vi "test Deploy with Module Already Reserved.vi"(8 "error in (no error)":errorcluster, 11 "TestCase in":refnum<class "SLSC Switch System Tests.lvclass">) -> (0 "error out":errorcluster, 3 "TestCase out":refnum<class "SLSC Switch System Tests.lvclass">)   [LabVIEW 2019, in "SLSC Switch System Tests.lvclass"]
uses:
  SLSC Switch System Tests.lvclass
  <vilib>/addons/_JKI Toolkits/VI Tester/TestCase.llb/TestCase.lvclass
  <vilib>/NI/VeriStand Custom Device Testing Tools/VeriStandTestCase/VeriStandTestCase.lvclass
  <vilib>/SLSC/SLSC.lvlib
  <vilib>/SLSC/Initialize Session with Devices.vi
  <vilib>/SLSC/Close Session.vi
  C:/Dev/GitHub/niveristand-custom-device-testing-tools/VeriStandTestCase/VeriStandTestCase.lvclass
  C:/Program Files (x86)/National Instruments/LabVIEW 2019/vi.lib/addons/_JKI Toolkits/VI Tester/TestCase.llb/TestCase.lvclass
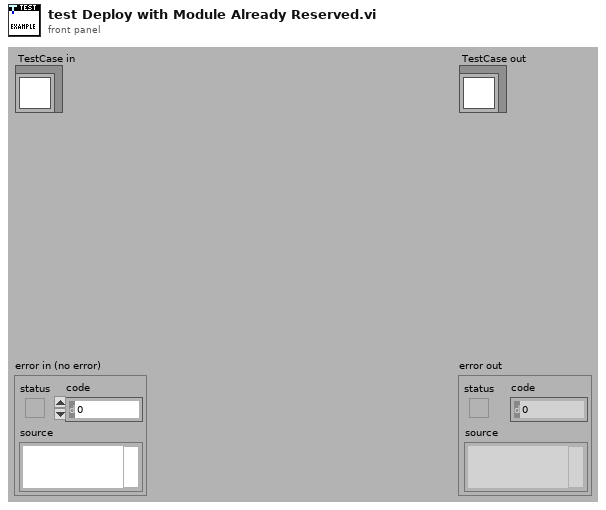
[diagram p1: front panel]
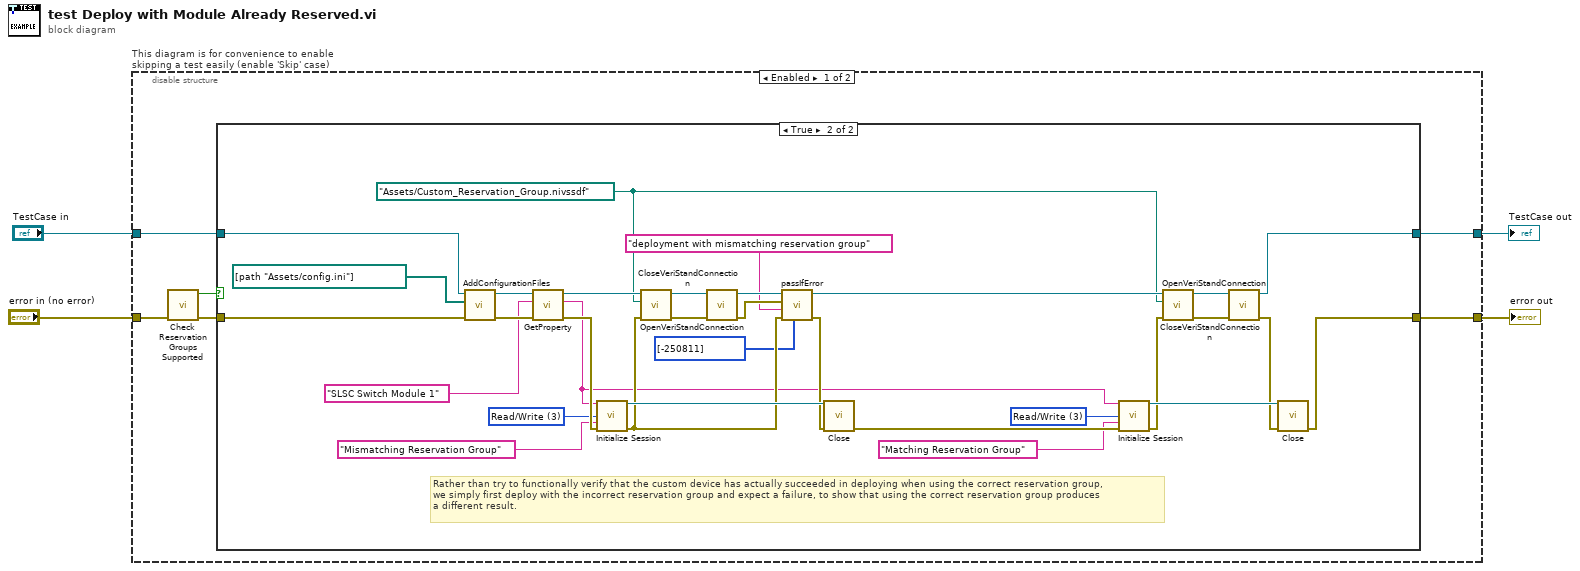
[diagram p0: block diagram]
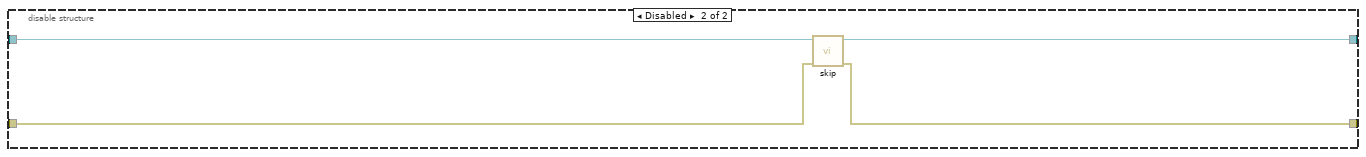
[diagram p3: hidden frame]
diagram:
  n1 = disable-structure "This diagram is for convenience to enable skipping a test easily (enable 'Skip' case)" shown="Enabled" {
    disable-tunnel: "TestCase in" -> [w10 w48]
    disable-tunnel: [w9 w46] -> w1
    disable-tunnel: [w8 w47] -> w3
    disable-tunnel: "error in (no error)" -> [w7 w45]
    frame Enabled {
      n2 = call "Check Reservation Groups Supported.vi"("error in"=w7) -> ("error out"=w6:errorcluster, "use reservation groups?"=w5:bool)  [unwired: 9 in]
      n3 = case shown="True" w5 {
        tunnel: w6 -> [w12 w41]
        tunnel: w10 -> [w11 w40]
        tunnel: [w11 w23] -> w9
        tunnel: [w12 w16] -> w8
        frame False {
        }
        frame True {
          w25 = 3 items=["None"=0, "Read Only"=1, "Read/Write"=3] ("reservation access (Read/Write)")
          w15 = path "Assets/Custom_Reservation_Group.nivssdf" ("overrides files")
          w34 = 3 items=["None"=0, "Read Only"=1, "Read/Write"=3] ("reservation access (Read/Write)")
          # "Rather than try to functionally verify that the custom device has actually succeeded in deploying when using the correct reservation group,\nwe simply first deploy with the incorrect reservation group and expect a failure, to show that using the correct reservation group produces\na different result."
          n4 = call <vilib>:"AddConfigurationFiles.vi"("error in (no error)"=w41, "configuration files"=path[] [path "Assets/config.ini"], "VeriStandTestCase in"=w40) -> ("error out"=w37:errorcluster, "VeriStandTestCase out"=w38:refnum<class "SLSC Switch System Tests.lvclass">)  [unwired: 7 in]
          n5 = call <vilib>:"GetProperty.vi"("error in (no error)"=w37, "key"="SLSC Switch Module 1", "VeriStandTestCase in"=w38) -> ("error out"=w44:errorcluster, "value"=w14:string, "VeriStandTestCase out"=w36:refnum<class "SLSC Switch System Tests.lvclass">)  [unwired: 6 in]
          n6 = call-poly <vilib>:"Initialize Session.vi"("devices"=w14, "reservation access (Read/Write)"=w34, "reservation group"="Mismatching Reservation Group", "error in (no error)"=w44) -> ("session out"=w32:refnum<k21>, "error out"=w18:errorcluster)  [unwired: 10 in]
          n7 = call-dynamic "OpenVeriStandConnection.vi"("error in (no error)"=w18, "System Definition File"=w15, "VeriStand Test Case in"=w36) -> ("error out"=w43:errorcluster, "VeriStand Test Case out"=w42:refnum<class "SLSC Switch System Tests.lvclass">)  [unwired: 6 in, 1 out]
          n8 = call-dynamic "CloseVeriStandConnection.vi"("error in (no error)"=w43, "VeriStand Test Case in"=w42) -> ("error out"=w20:errorcluster, "VeriStand Test Case out"=w22:refnum<class "SLSC Switch System Tests.lvclass">)  [unwired: 8 in]
          n9 = call-dynamic "passIfError.vi"("passing error codes (default = any error code)"=i32[] [-250811], "error in (no error)"=w18, "task (\"\")"="deployment with mismatching reservation group" ("task (\"\")"), "error"=w20, "TestCase in"=w22) -> ("error out"=w19:errorcluster, "TestCase out"=w21:refnum<class "SLSC Switch System Tests.lvclass">)  [unwired: 5 in]
          n10 = call-poly <vilib>:"Close.vi"("session in"=w32, "error in (no error)"=w19) -> ("error out"=w26:errorcluster)  [unwired: 13 in]
          n11 = call-poly <vilib>:"Initialize Session.vi"("devices"=w14, "reservation access (Read/Write)"=w25, "reservation group"="Matching Reservation Group", "error in (no error)"=w26) -> ("session out"=w31:refnum<k21>, "error out"=w29:errorcluster)  [unwired: 10 in]
          n12 = call-dynamic "OpenVeriStandConnection.vi"("error in (no error)"=w29, "System Definition File"=w15, "VeriStand Test Case in"=w21) -> ("error out"=w27:errorcluster, "VeriStand Test Case out"=w28:refnum<class "SLSC Switch System Tests.lvclass">)  [unwired: 6 in, 1 out]
          n13 = call-dynamic "CloseVeriStandConnection.vi"("error in (no error)"=w27, "VeriStand Test Case in"=w28) -> ("error out"=w30:errorcluster, "VeriStand Test Case out"=w23:refnum<class "SLSC Switch System Tests.lvclass">)  [unwired: 8 in]
          n14 = call-poly <vilib>:"Close.vi"("session in"=w31, "error in (no error)"=w30) -> ("error out"=w16:errorcluster)  [unwired: 13 in]
        }
      }
    }
    frame Disabled {
      n15 = call <vilib>:"skip.vi"("error in (no error)"=w45, "TestCase in"=w48) -> ("error out"=w47:errorcluster, "TestCase out"=w46:refnum<class "SLSC Switch System Tests.lvclass">)  [unwired: 8 in]
    }
  }
  "error out" <- w3
  "TestCase out" <- w1
